vi "Magnitude Square of Complex Number.vi"(5 "Real":fxp<+/-,18,1>, 7 "Imaginary":fxp<+/-,18,1>, 9 "Input Valid":bool=TRUE) -> (6 "Magnitude^2":fxp<+,48,14> format="%.39g", 10 "Output Valid":bool)   [LabVIEW 2011]
doc: "This VI computes the magnitude of a complex number using two DSP48E blocks in cascade fashion.\n\n<b> Latency = 6 Ticks </b>"
uses:
  <vilib>/rvi/FXPMathLib/basic elements/DSP48E/simVIs/niFpgaDsp48eRegisters.ctl
  <vilib>/rvi/FXPMathLib/basic elements/DSP48E/simVIs/niFpgaDsp48eEnables.ctl
  <vilib>/rvi/FXPMathLib/basic elements/DSP48E/simVIs/niFpgaDsp48eResets.ctl
  <vilib>/rvi/FXPMathLib/basic elements/DSP48E/simVIs/niFpgaDsp48eSimulationState.ctl
  <vilib>/rvi/FXPMathLib/basic elements/DSP48E/subVIs/niFpgaDsp48eType.ctl
  <vilib>/rvi/FXPMathLib/basic elements/DSP48E/subVIs/niFpgaDsp48eAlumodeOpmodeCarryinselState.ctl
  <vilib>/rvi/FXPMathLib/basic elements/DSP48E/subVIs/niFpgaDsp48eUseMultiplierState.ctl
  <vilib>/rvi/FXPMathLib/basic elements/DSP48E/subVIs/niFpgaDsp48eLogicUnitModeState.ctl
  <vilib>/rvi/FXPMathLib/basic elements/DSP48E/subVIs/niFpgaDsp48eSelectPatternState.ctl
  <vilib>/rvi/FXPMathLib/basic elements/DSP48E/subVIs/niFpgaDsp48eSelectMaskState.ctl
  <vilib>/rvi/FXPMathLib/basic elements/DSP48E/subVIs/niFpgaDsp48eAutoresetState.ctl
  <vilib>/rvi/FXPMathLib/basic elements/DSP48E/simVIs/niFpgaDsp48eSimMultiplier.vi
  <vilib>/rvi/FXPMathLib/basic elements/DSP48E/simVIs/niFpgaDsp48eSimArithmetic.vi
  <vilib>/rvi/FXPMathLib/basic elements/DSP48E/simVIs/niFpgaDsp48eSimPatternDetect.vi
  <vilib>/rvi/FXPMathLib/basic elements/DSP48E/simVIs/niFpgaDsp48eSimP.vi
  <vilib>/rvi/FXPMathLib/basic elements/DSP48E/simVIs/niFpgaDsp48eSimUpdateState.vi
  <vilib>/rvi/FXPMathLib/basic elements/DSP48E/simVIs/niFpgaDsp48eCheckMode.vi
  <vilib>/rvi/FXPMathLib/basic elements/DSP48E/simVIs/niFpgaDsp48eReportInvalidMode.vi
  <vilib>/rvi/FXPMathLib/basic elements/FxpDiscreteDelay/XNode/nifxpmath_DiscreteDelay.xnode
  <vilib>/rvi/FXPMathLib/FxpInterpret/XNode/nifxpmath_Interpret.xnode
  <vilib>/rvi/FXPMathLib/basic elements/DSP48E/XNode/niFpgaDsp48e.xnode
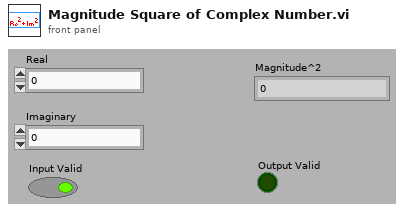
[diagram p1: front panel]
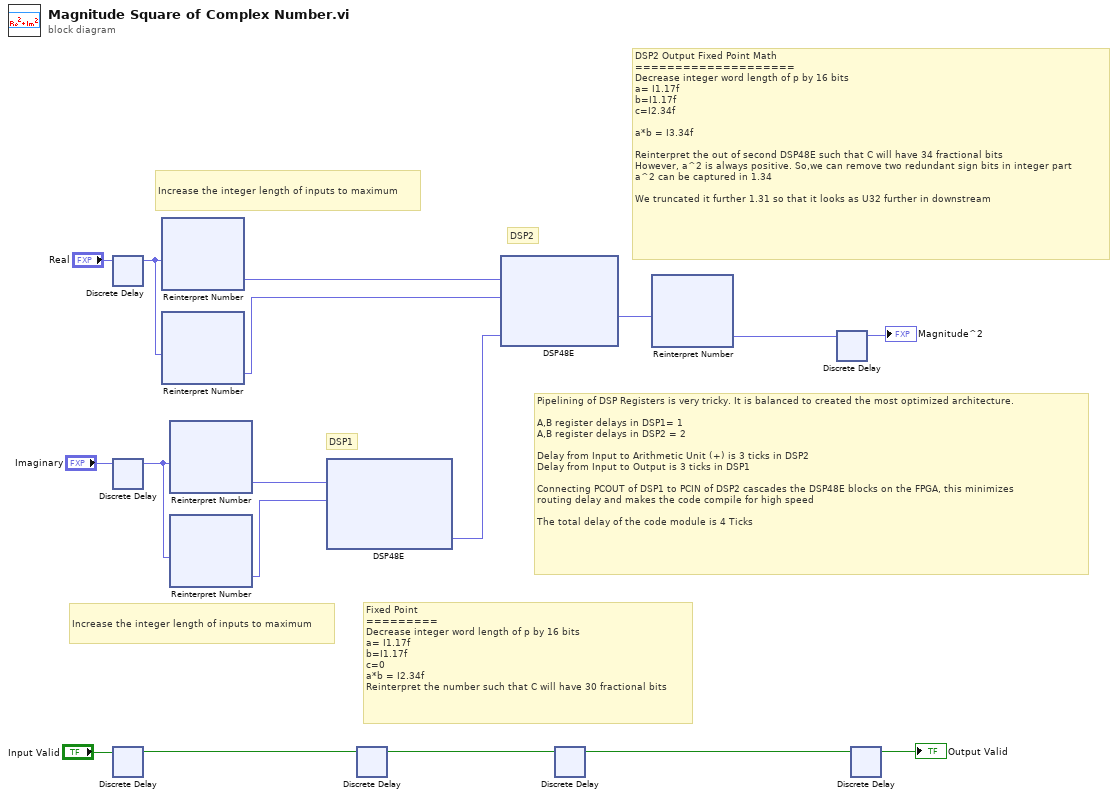
[diagram p0: block diagram]
diagram:
  # "Increase the integer length of inputs to maximum"
  # "DSP2"
  # "DSP1"
  # "Pipelining of DSP Registers is very tricky. It is balanced to created the most optimized architecture.\n\nA,B register delays in DSP1= 1\nA,B register delays in DSP2 = 2\n\nDelay from Input to Arithmetic Unit (+) is 3 ticks in DSP2\nDelay from Input to Output is 3 ticks in DSP1\n\nConnecting PCOUT of DSP1 to PCIN of DSP2 cascades the DSP48E blocks on the FPGA, this minimizes\nrouting delay and makes the code compile for high speed\n\nThe total delay of the code module is 4 Ticks"
  # "DSP2 Output Fixed Point Math\n====================\nDecrease integer word length of p by 16 bits\na= I1.17f\nb=I1.17f\nc=I2.34f\n\na*b = I3.34f\n\nReinterpret the out of second DSP48E such that C will have 34 fractional bits\nHowever, a^2 is always positive. So,we can remove two redundant sign bits in integer part\na^2 can be captured in 1.34\n\nWe truncated it further 1.31 so that it looks as U32 further in downstream"
  # "Increase the integer length of inputs to maximum"
  # "Fixed Point\n=========\nDecrease integer word length of p by 16 bits\na= I1.17f\nb=I1.17f\nc=0\na*b = I2.34f\nReinterpret the number such that C will have 30 fractional bits"
  n1 = xnode "Discrete Delay"("D"="Real") -> ("Q"=w3:fxp<+/-,18,1>)
  n2 = xnode "Discrete Delay"("D"="Imaginary") -> ("Q"=w4:fxp<+/-,18,1>)
  n3 = xnode "Discrete Delay"("D"="Input Valid") -> ("Q"=w2:bool)
  n4 = xnode "Reinterpret Number"("x"=w3) -> ("y"=w12:fxp<+/-,18,18>)
  n5 = xnode "Reinterpret Number"("x"=w3) -> ("y"=w13:fxp<+/-,18,18>)
  n6 = xnode "Reinterpret Number"("x"=w4) -> ("y"=w17:fxp<+/-,18,18>)
  n7 = xnode "Reinterpret Number"("x"=w4) -> ("y"=w16:fxp<+/-,18,18>)
  n8 = xnode "DSP48E"("a"=w17, "b"=w16) -> ("pcout"=w10:fxp<+/-,48,48>)  [unwired: 1 out]
  n9 = xnode "Discrete Delay"("D"=w2) -> ("Q"=w9:bool)
  n10 = xnode "DSP48E"("a"=w12, "b"=w13, "pcin"=w10) -> ("p"=w11:fxp<+/-,48,48>)
  n11 = xnode "Discrete Delay"("D"=w9) -> ("Q"=w7:bool)
  n12 = xnode "Reinterpret Number"("x"=w11) -> ("y"=w1:fxp<+,48,14>)
  n13 = xnode "Discrete Delay"("D"=w1) -> ("Q"=→"Magnitude^2":fxp<+,48,14>)
  n14 = xnode "Discrete Delay"("D"=w7) -> ("Q"=→"Output Valid":bool)
